vi "Pan_Head.vi"(2 "node":string, 3 "error in":errorcluster, 4 "speed":i32=40, 5 "target":sgl) -> (0 "error out":errorcluster)   [LabVIEW 2013]
doc: "This will nod the head."
uses:
  ROS/MessageBuilding/Primitives/subs/float32Scalar.vi
  ROS/MessageBuilding/Primitives/subs/i32Scalar.vi
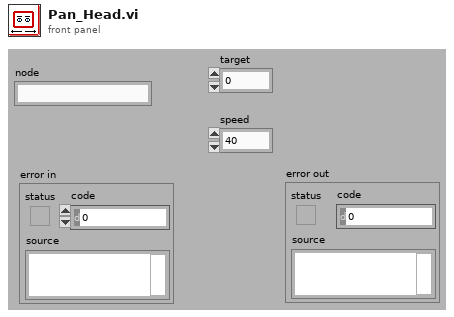
[diagram p1: front panel]
types:
  T1 = typedef "_ROSControl.ctl" = cluster{"topic port":u16, "Node":string, "topic":string, "type":string, "node port":u32, "error ":errorcluster, "Direction":T2, "APIs":string[]}
  T2 = typedef "_ROSDirection.ctl" = enum16{"Node", "Publisher", "Subscriber", "Service Client"}
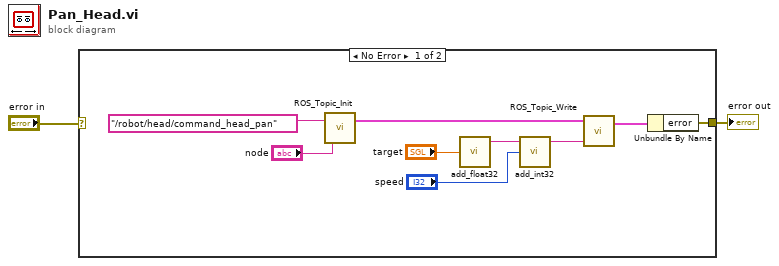
[diagram p0: block diagram]
diagram:
  n1 = case shown="No Error" "error in" {
    selector: "error in" -> [_ w12]
    tunnel: [w9 w12] -> w2
    frame No Error {
      n2 = call "ROS_Topic_Init.vi"("node"="node", "topic"="/robot/head/command_head_pan") -> ("ROS out"=w7:T1)  [unwired: 1 in]
      n3 = call-poly "add_float32.vi"("Numeric"="target") -> ("msg out"=w4:string)  [unwired: 4 in]
      n4 = call-poly "add_int32.vi"("Numeric"="speed", "msg in"=w4) -> ("msg out"=w3:string)  [unwired: 3 in]
      n5 = call "ROS_Topic_Write.vi"("Msg in"=w3, "ROS in"=w7) -> ("ROS out"=w10:T1)  [unwired: 2 in]
      n6 = Unbundle By Name(w10) -> ("error"=w9:errorcluster)
    }
    frame Error {
    }
  }
  "error out" <- w2
